vi "Estimate Velocity from Transforms.vi"(8 "error in (no error)":errorcluster, 10 "velocity transform vector in":dbl[](array[numeric]), 11 "velocity transform matrix in":T1) -> (0 "error out":errorcluster, 3 "estimated steering frame velocity":dbl[](array[numeric]))   [LabVIEW 2017, in "NI_Robotics_Steering Frame.lvclass"]
uses:
  <vilib>/robotics/Steering/Steering Frame/NI_Robotics_Steering Frame.lvclass
  <vilib>/Analysis/Matrix/Datatypes/RealMatrix.ctl
  <vilib>/robotics/Utilities/NI_Robotics Utilities.lvlib
  <vilib>/Analysis/NI_AALPro.lvlib
  <vilib>/Analysis/Matrix/NI_Matrix.lvlib
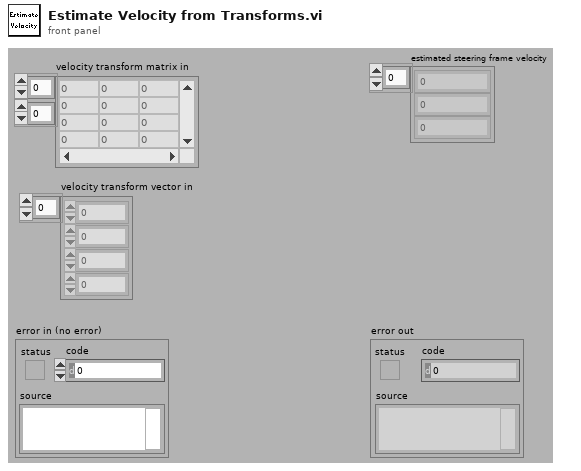
[diagram p1: front panel]
types:
  T1 = typedef "NI_Matrix.lvlib/RealMatrix.ctl" = dbl[][]
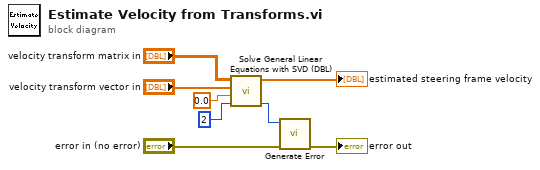
[diagram p0: block diagram]
diagram:
  n1 = call <vilib>:"Solve General Linear Equations with SVD (DBL).vi"("iteration"=2, "relative tolerance"=0.0, "Known Vector"="velocity transform vector in", "Input Matrix"="velocity transform matrix in") -> ("error"=w1:i32, "Solution Vector"=→"estimated steering frame velocity":dbl[])  [unwired: 6 in]
  n2 = call <vilib>:"Generate Error.vi"("error in (no error)"="error in (no error)", "code"=w1) -> ("error out"=→"error out":errorcluster)  [unwired: 9 in]
